vi "Set Splitter Position.vi"(6 "Splitter Position":i32, 8 "error in (no error)":errorcluster, 10 "Limits":cluster{"Left":i16, "Right":i16}, 11 "Interaction Splitter in":refnum<class "Interaction Splitter.lvclass">) -> (0 "error out":errorcluster, 3 "Interaction Splitter out":refnum<class "Interaction Splitter.lvclass">)   [LabVIEW 2021, in "Interaction Splitter.lvclass"]
doc: "Copyright 2018, Wiebe Walstra, wiebe@carya.nl."
uses:
  Interaction Splitter.lvclass
  Interaction Splitter.lvclass/Interaction Splitter.ctl
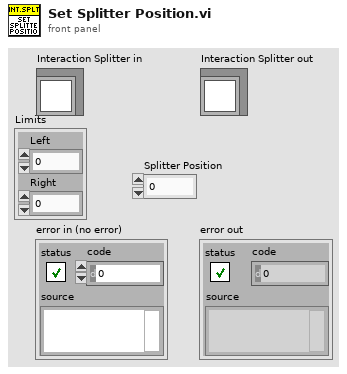
[diagram p1: front panel]
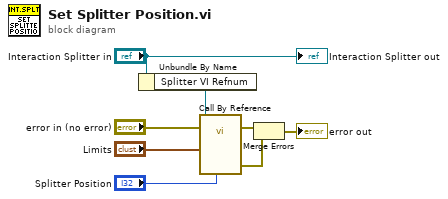
[diagram p0: block diagram]
diagram:
  n1 = Unbundle By Name("Interaction Splitter in") -> ("Splitter VI Refnum"=w1:refnum<vi>)
  n2 = call-by-ref "?"(reference=w1, error in="error in (no error)", "Splitter Position"="Splitter Position", "Limits"="Limits") -> (error out=w6:errorcluster, 0:"error out"=w2:errorcluster)  [unwired: 9 in, 1 out]
  n3 = Merge Errors(w6, w2) -> (→"error out":errorcluster)
  "Interaction Splitter out" <- "Interaction Splitter in"
